vi "youtube_demo.vi"() -> ()   [LabVIEW 2020]
uses:
  <vilib>/Analysis/2dsp.llb/Real FFT.vi
  <vilib>/express/express analysis/Spectral/Block/exnSpectralBlock spectral measurements power poly.vi
  <vilib>/express/express analysis/Spectral/Block/exnSpectralBlock spectral measurements power WFM.vi
  <vilib>/addons/control/pid/pid.llb/PID Advanced (DBL).vi
  <vilib>/addons/control/pid/pid.llb/PID (DBL).vi
  <vilib>/express/express analysis/Spectral/XNode/ExpressSpectralMeasurementsBlockNode.xnode
  <vilib>/Analysis/NI_AALPro.lvlib
  <vilib>/gmath/NI_Gmath.lvlib
  <vilib>/addons/control/pid/NI_PID_pid.lvlib
panel:
  out "Waveform Graph":dbl[](graph)
  out "Time Domain Plot":dbl[](graph)
  out "Laplace {X}":dbl[](array[numeric])
  in  "Time Domain Array":dbl[](array[numeric])
  out "Power Spectrum (non normalised manual)":cluster{"X":dbl, "Y":dbl}[](graph)
  out "power array (normalised)":dbl[](array[numeric])
  out "Amplitude LHS of FFT vs Frequency (Hz)":cluster{"X":dbl, "Y":dbl}[](graph)
  out "LHS of FFT array":cdb[](array[numeric])
  out "frequency Array":dbl[](array[numeric])
  out "index array":dbl[](array[numeric])
  out "initialized array":dbl[](array[numeric])
  in  "Graphs":T1(tab)
  out "Power Spectrum":cluster{"f0":dbl, "df":dbl, "magnitude":dbl[]}(graph)
  in  "path":path
  out "This is My Audio Graph":waveform(dbl)[](graph)
  out "Waveform Chart":waveform(dbl)[](graph)
  out "Fast Fourier Transform":dbl[](graph)
  in  "FFT size (how many samples to take)":i32=-1
  out "FFT size":i32
  in  "Waveform Data":T2(tab)
  out "When does my waveform start":timestamp
  out "Sampling Time Interval (s)":dbl
  out "Data Values from WaveForm":dbl[](array[numeric])
  out "Sampling Frequency (Hz)":dbl
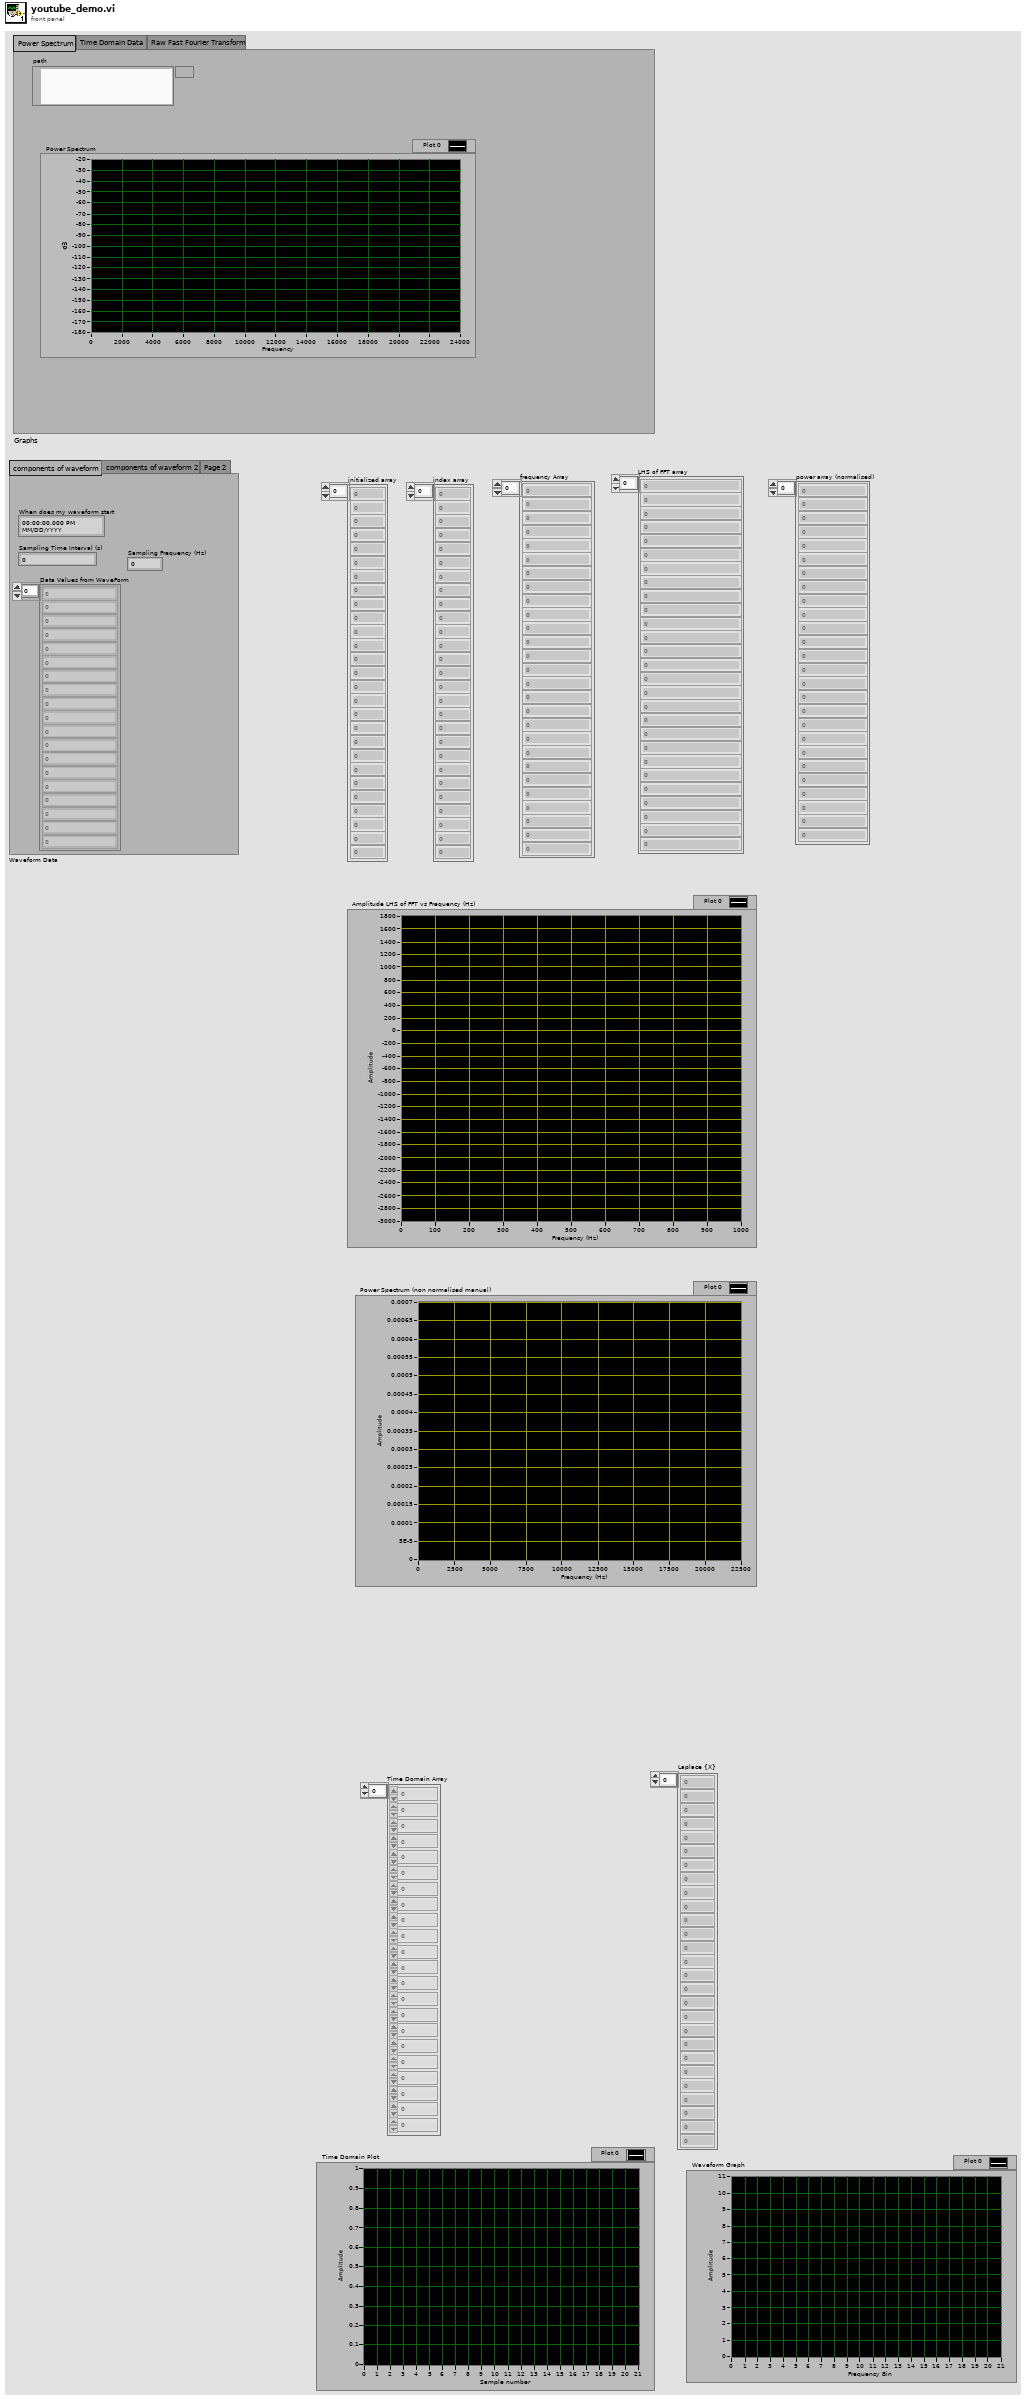
[diagram p1: front panel]
types:
  T1 = enum32{"Power Spectrum", "Time Domain Data", "Raw Fast Fourier Transform"}
  T2 = enum32{"components of waveform", "components of waveform 2", "Page 2"}
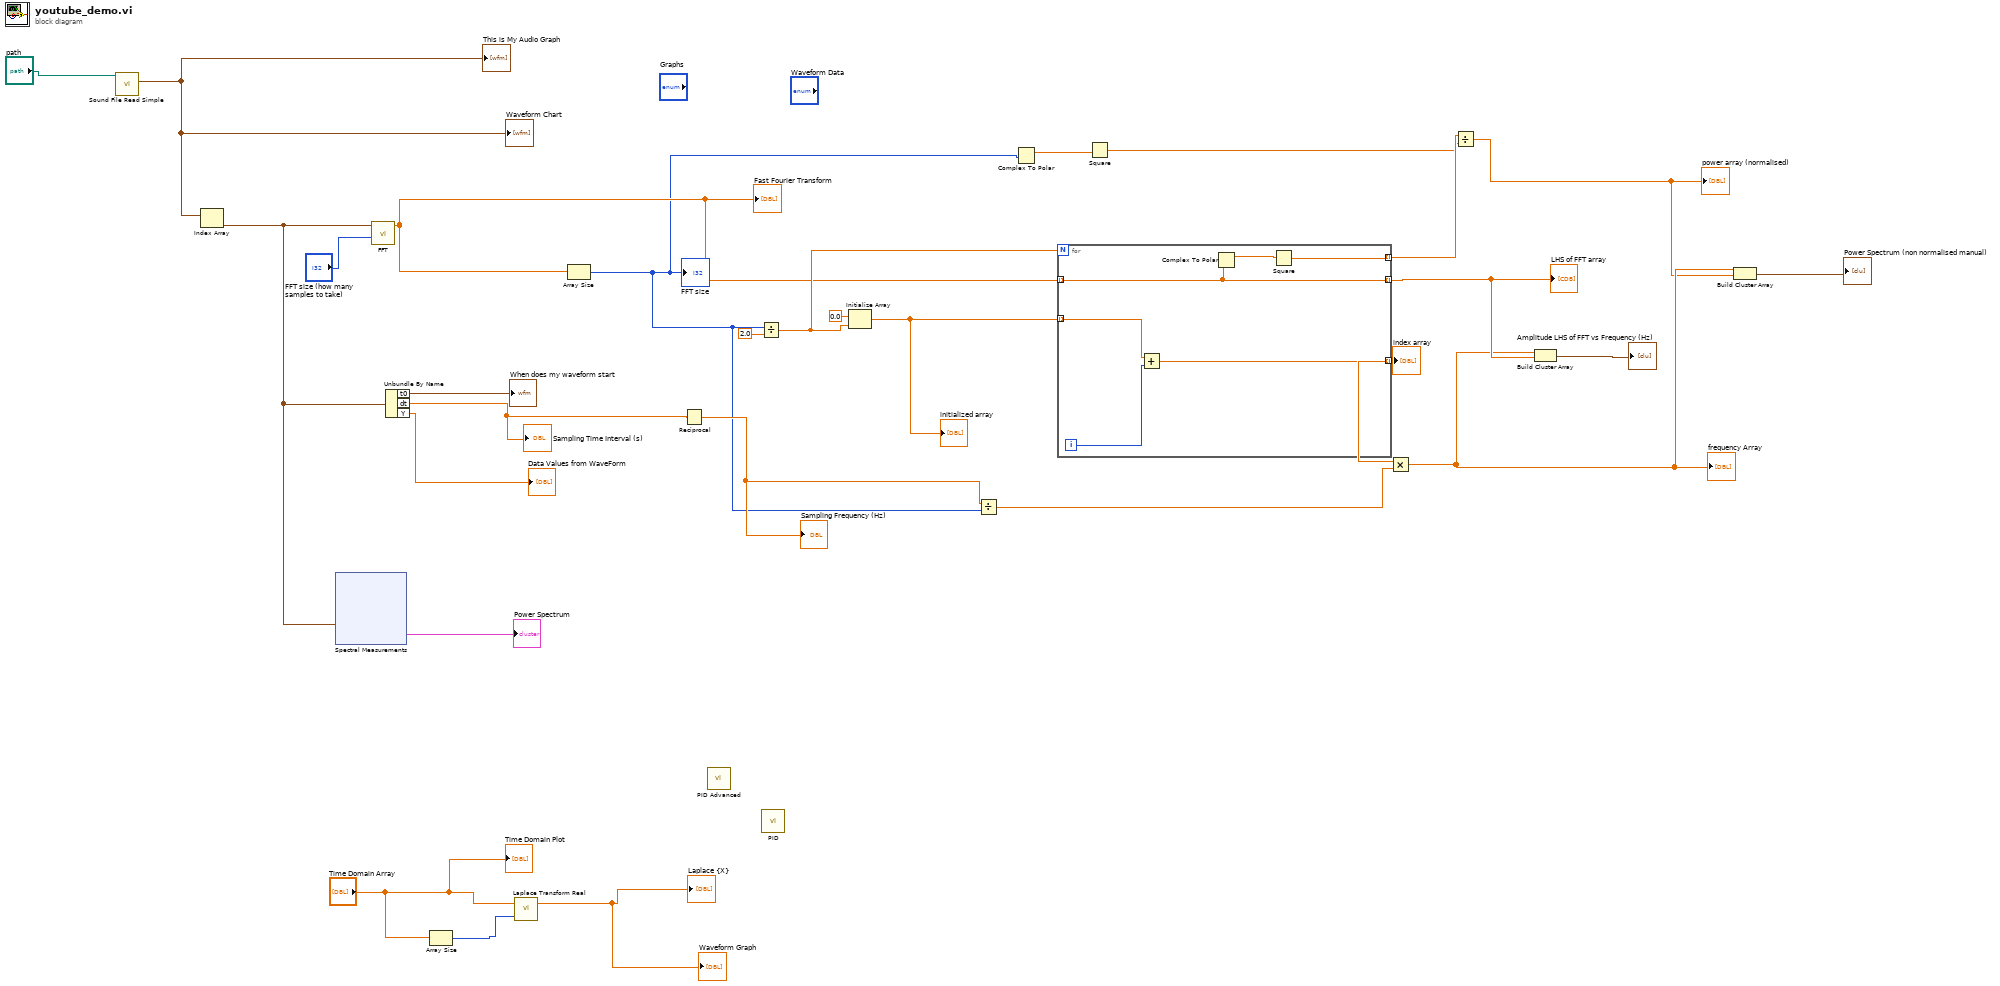
[diagram p0: block diagram]
diagram:
  n1 = call <vilib>:"Sound File Read Simple.vi"("path"="path") -> ("data"=w25:waveform(dbl)[])  [unwired: 7 in, 3 out]
  "This is My Audio Graph" <- w25
  "Waveform Chart" <- w25
  n2 = Index Array(array=w25) -> (element=w24:waveform(dbl))  [unwired: 1 in]
  n3 = xnode "Spectral Measurements"("Signals"=w24) -> ("Power Spectrum"=→"Power Spectrum":cluster{"f0":dbl, "df":dbl, "magnitude":dbl[]})  [unwired: 1 in, 1 out]
  n4 = call-poly <vilib>:"FFT.vi"("FFT size"="FFT size (how many samples to take)", "X"=w24) -> ("FFT {X}"=w13:cdb[])  [unwired: 8 in, 1 out]
  "Fast Fourier Transform" <- w13
  n5 = Unbundle By Name(w24) -> ("t0"=→"When does my waveform start":timestamp, "dt"=w17:dbl, "Y"=→"Data Values from WaveForm":dbl[])
  "Sampling Time Interval (s)" <- w17
  n6 = Array Size(array="Time Domain Array") -> (size(s)=w3:i32)
  n7 = call <vilib>:"Laplace Transform Real.vi"("end"=w3, "X"="Time Domain Array") -> ("Laplace {X}"=→"Laplace {X}" →"Waveform Graph":dbl[])  [unwired: 1 out]
  n8 = Array Size(array=w13) -> (size(s)=w8:i32)
  "FFT size" <- w8
  n9 = Reciprocal(x=w17) -> (1/x=w16:dbl)
  "Sampling Frequency (Hz)" <- w16
  n10 = call-poly <vilib>:"PID Advanced.vi"() -> ()  [unwired: 14 in, 2 out]
  n11 = Divide(x=w8, y=2.0) -> (x/y=w19:dbl)
  n12 = call-poly <vilib>:"PID.vi"() -> ()  [unwired: 10 in, 2 out]
  n13 = Initialize Array(0.0 ("element"), w19) -> (w18:dbl[])
  "initialized array" <- w18
  n14 = Divide(x=w16, y=w8) -> (x/y=w14:dbl)
  n15 = Complex To Polar(r * e^(i*theta)=w8) -> (r=w7:dbl)  [unwired: 1 out]
  n16 = for {
    N: w19 -> [_]
    tunnel: w18 -> [w34] mode=indexing
    tunnel: [w32] -> w15 mode=indexing
    tunnel: w13 -> [w31] mode=indexing
    tunnel: [w31] -> w11 mode=indexing
    tunnel: [w29] -> w6 mode=indexing
    i -> [w33]
    n17 = Add(x=w34, y=w33) -> (x+y=w32:dbl)
    n18 = Complex To Polar(r * e^(i*theta)=w31) -> (r=w30:dbl)  [unwired: 1 out]
    n19 = Square(x=w30) -> (x^2=w29:dbl)
  }
  "index array" <- w15
  "LHS of FFT array" <- w11
  n20 = Square(x=w7) -> (x^2=w5:dbl)
  n21 = Multiply(x=w15, y=w14) -> (x*y=w10:dbl[])
  "frequency Array" <- w10
  n22 = Divide(x=w6, y=w5) -> (x/y=w4:dbl[])
  "power array (normalised)" <- w4
  n23 = Build Cluster Array(w10, w11) -> (→"Amplitude LHS of FFT vs Frequency (Hz)":cluster{dbl, cdb}[])
  n24 = Build Cluster Array(w10, w4) -> (→"Power Spectrum (non normalised manual)":cluster{dbl, dbl}[])
  "Time Domain Plot" <- "Time Domain Array"
